vi "Check Angle.vi"(7 "memory value":u16, 11 "state data in":T1) -> (2 ">=edge 1":bool, 3 "state data out":T1)   [LabVIEW 2015, in "Engine Simulation Toolkit.lvlib" / "Digital Pattern Generation.lvlib"]
uses:
  Digital Pattern Generation.lvlib
  state data.ctl
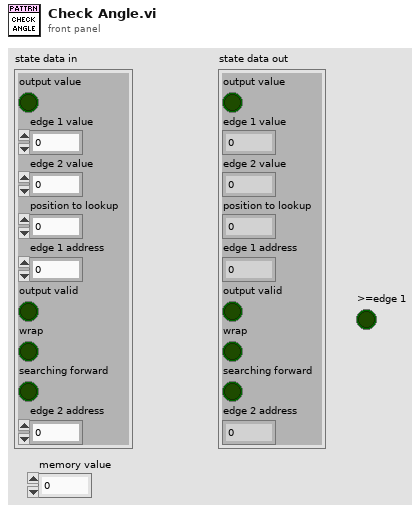
[diagram p1: front panel]
types:
  T1 = typedef "Engine Simulation Toolkit.lvlib/Digital Pattern Generation.lvlib/state data.ctl" = cluster{"output value":bool, "edge 1 value":u16, "edge 2 value":u16, "position to lookup":u16, "edge 1 address":fxp<+,11,11>, "output valid":bool, "wrap":bool, "searching forward":bool, "edge 2 address":fxp<+,11,11>}
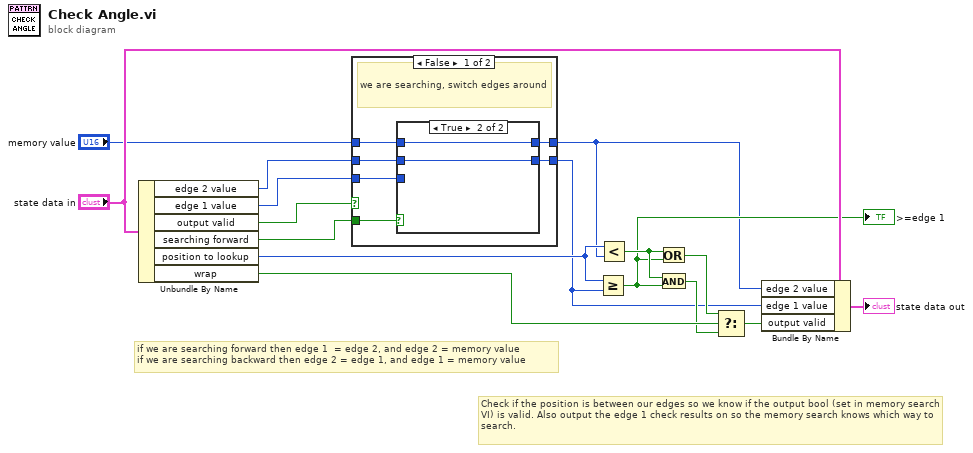
[diagram p0: block diagram]
diagram:
  # "if we are searching forward then edge 1  = edge 2, and edge 2 = memory value\nif we are searching backward then edge 2 = edge 1, and edge 1 = memory value"
  # "Check if the position is between our edges so we know if the output bool (set in memory search VI) is valid. Also output the edge 1 check results on so the memory search knows which way to search."
  n1 = Unbundle By Name("state data in") -> ("edge 2 value"=w2:u16, "edge 1 value"=w1:u16, "output valid"=w3:bool, "searching forward"=w8:bool, "position to lookup"=w7:u16, "wrap"=w14:bool)
  n2 = case shown="False" w3 {
    tunnel: w8 -> [w22 _]
    tunnel: w2 -> [w21 w28]
    tunnel: w1 -> [w20 w27]
    tunnel: "memory value" -> [w19 _]
    tunnel: [w18 w27] -> w5
    tunnel: [w17 w28] -> w4
    frame False {
      # "we are searching, switch edges around"
      n3 = case shown="True" w22 {
        tunnel: w21 -> [_ w26]
        tunnel: w20 -> [w24 _]
        tunnel: [w23 w26] -> w18
        tunnel: w19 -> [w23 w25]
        tunnel: [w24 w25] -> w17
        frame False {
        }
        frame True {
        }
      }
    }
    frame True {
      # "First call or we are not searching, don't touch edges"
    }
  }
  n4 = Greater Or Equal?(x=w7, y=w5) -> (x >= y?=w9:bool)
  ">=edge 1" <- w9
  n5 = Less?(x=w7, y=w4) -> (x < y?=w10:bool)
  n6 = Or(x=w10, y=w9) -> (x .or. y?=w13:bool)
  n7 = And(x=w10, y=w9) -> (x .and. y?=w12:bool)
  n8 = Select(t=w13, s=w14, f=w12) -> (s? t:f=w11:bool)
  n9 = Bundle By Name(cluster="state data in", "edge 2 value"=w4, "edge 1 value"=w5, "output valid"=w11) -> (→"state data out":T1)
